vi "Arduino Controler.vi"   [LabVIEW 2018]
uses:
  <vilib>/LabVIEW Interface for Arduino/LabVIEW Interface for Arduino.lvlib
  <vilib>/LabVIEW Interface for Arduino/Type Defs/Board Type.ctl
  <vilib>/LabVIEW Interface for Arduino/Type Defs/Connection Type.ctl
types:
  T1 = typedef "LabVIEW Interface for Arduino.lvlib/Connection Type.ctl" = enum8{"USB / Serial", "XBEE", "BlueSmirf (Bluetooth)"}
  T2 = typedef "LabVIEW Interface for Arduino.lvlib/Board Type.ctl" = enum16{"Uno", "Dimuelanove w/Atmega 328", "Mega 2560"}
  T3 = typedef "LabVIEW Interface for Arduino.lvlib/Arduino Resource.ctl" = cluster{"VISA resource":refnum<visa-resource-name>, "Board Type":T2, "Connection Type":enum8{"USB / Serial"}, "Bytes Per Packet (15)":u8}
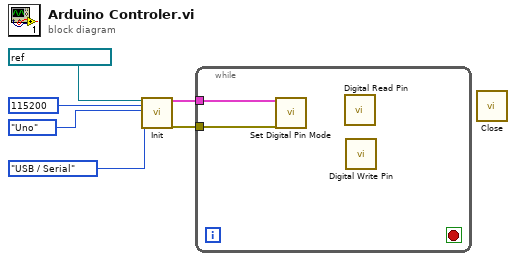
[diagram p0: block diagram]
diagram:
  n1 = call <vilib>:"Init.vi"("VISA resource"=refnum<visa-resource-name> "ASRL1::INSTR", "Baud Rate (115200)"=u32 115200, "Board Type (Uno)"=Board_Type."Uno", "Connection Type (USB/Serial)"=Connection_Type."USB / Serial") -> ("Arduino Resource"=w2:T3, "error out"=w1:errorcluster)  [unwired: 14 in]
  n2 = while {
    tunnel: w2 -> [w8]
    tunnel: w1 -> [w7]
    stop <- _ stop-if-true
    n3 = call <vilib>:"Set Digital Pin Mode.vi"("Arduino Resource"=w8, "error in"=w7) -> ()  [unwired: 12 in, 2 out]
    n4 = call <vilib>:"Digital Read Pin.vi"() -> ()  [unwired: 13 in, 3 out]
    n5 = call <vilib>:"Digital Write Pin.vi"() -> ()  [unwired: 14 in, 2 out]
  }
  n6 = call <vilib>:"Close.vi"() -> ()  [unwired: 15 in, 1 out]
